vi "case_caution.vi"() -> ()   [LabVIEW 2018]
panel:
  out "Numeric 2":dbl
  in  "Numeric":dbl
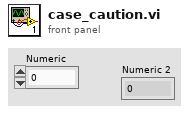
[diagram p1: front panel]
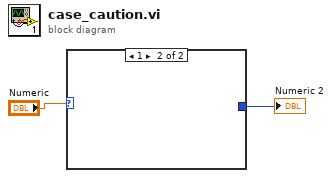
[diagram p0: block diagram]
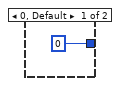
[diagram p2: hidden frame]
diagram:
  n1 = case shown="1" "Numeric" {
    tunnel: [0 _] -> w1
    frame 0, Default {
    }
    frame 1 {
    }
  }
  "Numeric 2" <- w1
